vi "Write Value.vi"(8 "error in (no error)":errorcluster caption="entrée d'erreur (pas d'erreur)", 10 "Data":string, 11 "DAQmxTask en entrée":refnum<class "DAQmxTask.lvclass">) -> (0 "error out":errorcluster caption="sortie d'erreur", 3 "DAQmxTask en sortie":refnum<class "DAQmxTask.lvclass">)   [LabVIEW 2019, in "DAQmxTask.lvclass"]
uses:
  DAQmxTask.lvclass
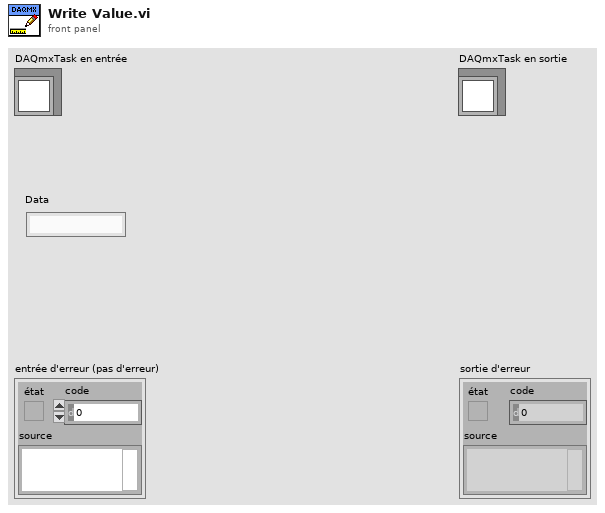
[diagram p1: front panel]
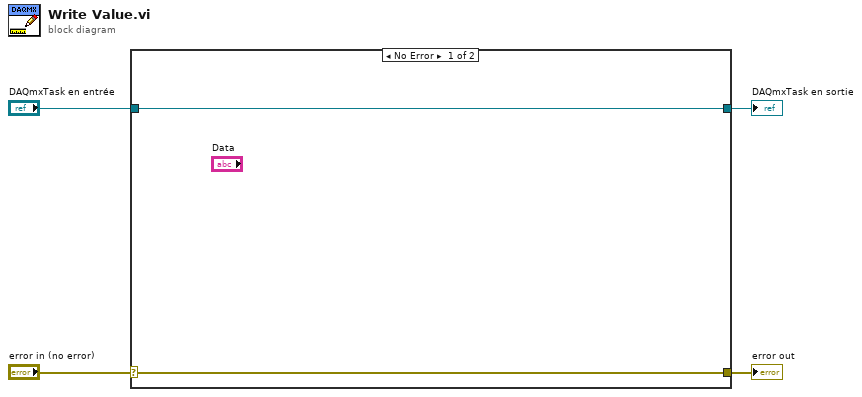
[diagram p0: block diagram]
diagram:
  n1 = case shown="No Error" "error in (no error)" {
    selector: "error in (no error)" -> [w5 w8]
    tunnel: [w5 w8] -> w3
    tunnel: [w6 w7] -> w1
    tunnel: "DAQmxTask en entrée" -> [w6 w7]
    frame No Error {
    }
    frame Error {
    }
  }
  "error out" <- w3
  "DAQmxTask en sortie" <- w1
